vi "Load and Vin SMU Measurement.vi"() -> ()   [LabVIEW 2021, in "Main.lvlib"]
doc: "Demonstrates how to use the DC Voltage Output Function to force an output voltage. This example initializes a session, configures the Output Function, Sense, Autorange, Voltage Level and Current Limit, initiates generation, waits for a specified delay, and measures the voltage and current output. This example uses Single Point source mode."
uses:
  Main.lvlib
  controls/DMM Meas Type.ctl
  controls/DMM Resolution.ctl
  controls/SMU Config.ctl
  controls/Current Meas.ctl
  DMM.lvlib
panel:
  out "Current Measurement":T1
  in  "SMU Config":T2={"Voltage Level"=2.0, "Current Limit"=0.01} {"Current Limit" format="%.3p"; "Voltage Level" format="%.5p"}
  in  "Tektronix Scope":refnum<visa-resource-name>
  in  "Load DMM":refnum<k15>="Dev1" caption="SMU DMM"
  in  "Load DMM":refnum<k15>="Dev1"
  out "Division Number":i32
  in  "Sample Rate":dbl=3125000000.0
  in  "Maximum Record Length":dbl=250000000.0 format="%#_6e"
  out "SMU Measurement":dbl format="%.6p"
  in  "SMU DMM Measurement":T3
  in  "SMU Resolution in Digits":T4=5.5 items=["3 1/2"=3.5, "4 1/2"=4.5, "5 1/2"=5.5, "6 1/2"=6.5, "7 1/2"=7.5]
  out "Load Voltage":dbl caption="SMU Measurement" format="%.6p"
  in  "Load DMM Measurement":T3 caption="SMU DMM Measurement"
  in  "Load SMU":refnum<k15>="Dev1"
  in  "Load SMU Channel":string="0"
  out "Load SMU Voltage":dbl
  in  "error in":errorcluster
  out "error out":errorcluster
  out "Voltage Measurement":dbl caption="Vin SMU Voltage"
  in  "Vin SMU Channel":string="0"
  in  "Vin SMU":refnum<k15>="Dev1"
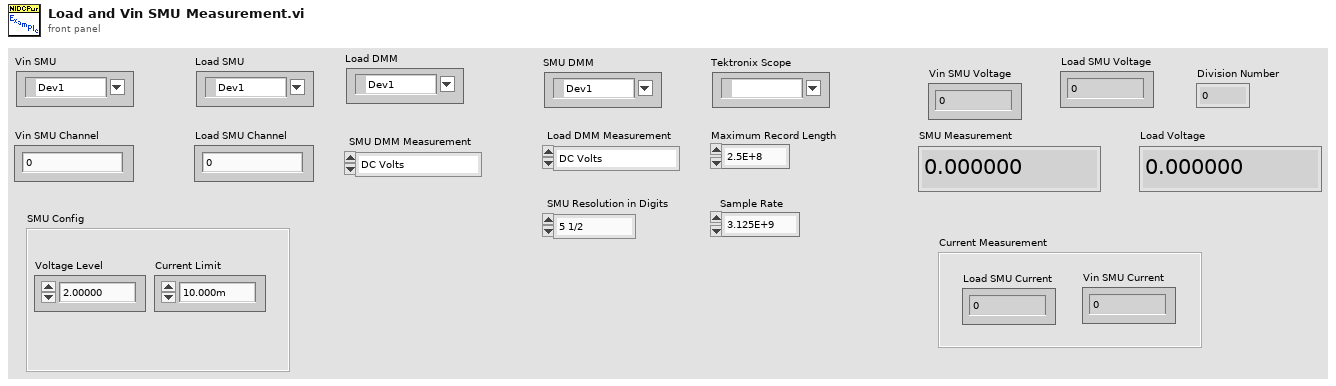
[diagram p1: front panel]
types:
  T1 = typedef "Main.lvlib/Current Meas.ctl" = cluster{"Load SMU Current":dbl, "Current Measurement":dbl}
  T2 = typedef "Main.lvlib/SMU Config.ctl" = cluster{"Voltage Level":dbl, "Current Limit":dbl}
  T3 = typedef "DMM.lvlib/DMM Meas Type.ctl" = enum16{"DC Volts", "AC Volts", "DC Current", "AC Current", "2-wire Resistance", "4-wire Resistance", "Diode", "Frequency", "Period", "AC Volts DC Coupled", "Capacitance", "Inductance", "Temperature"}
  T4 = typedef "DMM.lvlib/DMM Resolution.ctl" = dbl
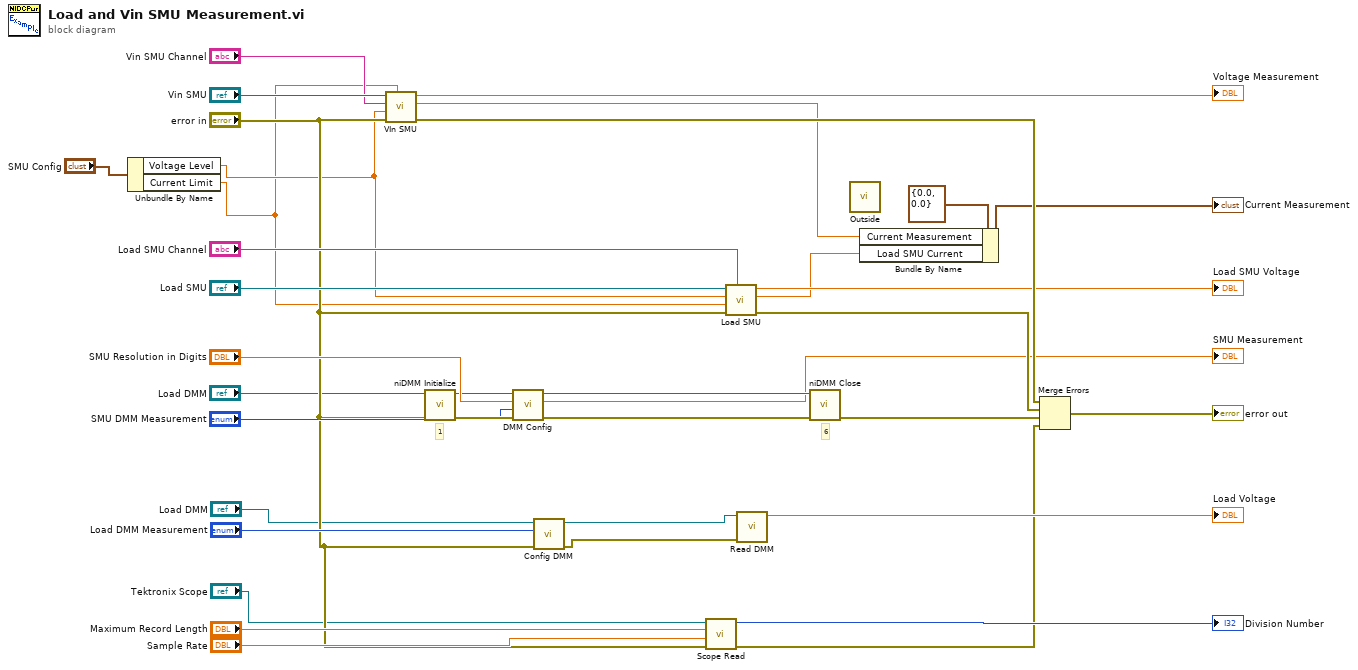
[diagram p0: block diagram]
diagram:
  # "1"
  # "6"
  n1 = Unbundle By Name("SMU Config") -> ("Voltage Level"=w6:dbl, "Current Limit"=w5:dbl)
  n2 = call "VIn SMU.vi"("Current Limit"=w5, "error in (no error)"="error in", "Voltage Level"=w6, "Vin SMU Channel"="Vin SMU Channel", "IVI Refnum in"="Vin SMU") -> ("error out"=w35:errorcluster, "Current Measurement"=w1:dbl, "Voltage Measurement"=→"Voltage Measurement":dbl)  [unwired: 4 in]
  n3 = call <instrlib>:"niDMM Initialize.vi"("error in (no error)"="error in", "Instrument Descriptor"="Load DMM") -> ("error out"=w21:errorcluster, "instrument handle out"=w22:refnum<k15>)  [unwired: 8 in]
  n4 = call "DMM Config.vi"("error in (no error)"=w21, "SMU DMM Measurement"="SMU DMM Measurement", "SMU Resolution in Digits"="SMU Resolution in Digits", "IVI Refnum in"=w22) -> ("error out"=w12:errorcluster, "Measurement"=→"SMU Measurement":dbl, "IVI Refnum out"=w23:refnum<k15>)  [unwired: 5 in]
  n5 = call "Config DMM.vi"("error in (no error)"="error in", "Load DMM Measurement"="Load DMM Measurement", "IVI Refnum in"="Load DMM") -> ("error out"=w28:errorcluster, "IVI Refnum out"=w27:refnum<k15>)  [unwired: 7 in]
  n6 = call "Scope Read.vi"("error in (no error)"="error in", "Sample Rate"="Sample Rate", "Maximum Record Length"="Maximum Record Length", "VISA Refnum in"="Tektronix Scope") -> ("error out"=w13:errorcluster, "Division Number"=→"Division Number":i32)  [unwired: 6 in]
  n7 = call "Load SMU.vi"("Load SMU Channel"="Load SMU Channel", "error in (no error)"="error in", "Current Limit"=w5, "Voltage Level"=w6, "IVI Refnum in"="Load SMU") -> ("error out"=w31:errorcluster, "Numeric"=w2:dbl, "Numeric 2"=→"Load SMU Voltage":dbl)  [unwired: 4 in]
  n8 = call "Read DMM.vi"("error in (no error)"=w28, "IVI Refnum in"=w27) -> ("Measurement"=→"Load Voltage":dbl)  [unwired: 9 in]
  n9 = call <instrlib>:"niDMM Close.vi"("error in (no error)"=w12, "instrument handle"=w23) -> ("error out"=w18:errorcluster)  [unwired: 9 in]
  n10 = call "Outside.vi"() -> ()  [unwired: 12 in]
  n11 = Bundle By Name(cluster=T1 {"Load SMU Current"=0.0, "Current Measurement"=0.0} ("Current Measurement"), "Current Measurement"=w1, "Load SMU Current"=w2) -> (→"Current Measurement":T1)
  n12 = Merge Errors(w35, w31, w18, w13) -> (→"error out":errorcluster)
